vi "DHE_GetShutdownMacro.vi"() -> (7 "DHE_InitMacro":path)   [LabVIEW 2016]
uses:
  private/vis/DHE_VarAction.ctl
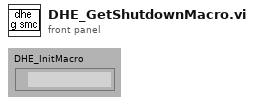
[diagram p1: front panel]
types:
  T1 = typedef "DHE_VarAction.ctl" = enum16{"read", "write"}
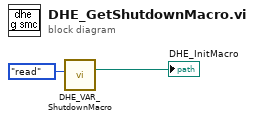
[diagram p0: block diagram]
diagram:
  n1 = call "DHE_VAR_ShutdownMacro.vi"("action"=DHE_VarAction."read") -> ("InstLibPath"=→"DHE_InitMacro":path)  [unwired: 1 in, 9 out]
